vi "Diff_Drive_System_Dash_Write.vi"   [LabVIEW 2019]
uses:
  Diff_Drive_System_Globals.vi
  <vilib>/Rock Robotics/Network Tables/NT Write Numeric Array.vi
  <vilib>/Rock Robotics/Network Tables/NT Write Number.vi
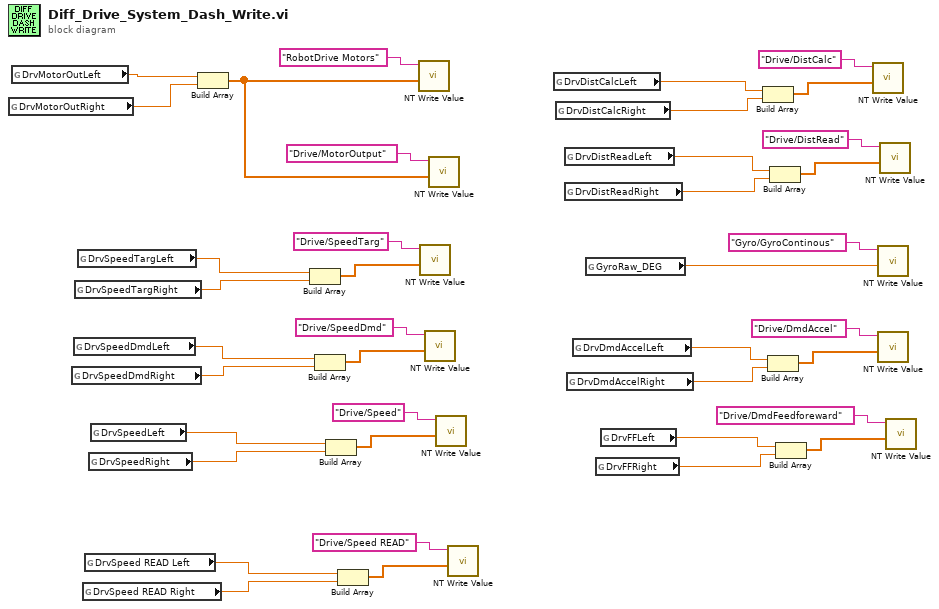
[diagram p0: block diagram]
diagram:
  n1 = global read "Diff_Drive_System_Globals.vi" "DrvMotorOutRight"() -> (w21:dbl)
  n2 = global read "Diff_Drive_System_Globals.vi" "DrvMotorOutLeft"() -> (w22:dbl)
  n3 = global read "Diff_Drive_System_Globals.vi" "DrvSpeedDmdRight"() -> (w16:dbl)
  n4 = global read "Diff_Drive_System_Globals.vi" "DrvSpeedDmdLeft"() -> (w17:dbl)
  n5 = global read "Diff_Drive_System_Globals.vi" "DrvSpeedTargRight"() -> (w18:dbl)
  n6 = global read "Diff_Drive_System_Globals.vi" "DrvSpeedTargLeft"() -> (w19:dbl)
  n7 = global read "Diff_Drive_System_Globals.vi" "DrvSpeed READ Right"() -> (w1:dbl)
  n8 = global read "Diff_Drive_System_Globals.vi" "DrvSpeed READ Left"() -> (w2:dbl)
  n9 = global read "Diff_Drive_System_Globals.vi" "DrvSpeedRight"() -> (w14:dbl)
  n10 = global read "Diff_Drive_System_Globals.vi" "DrvSpeedLeft"() -> (w15:dbl)
  n11 = Build Array(w22, w21) -> (w20:dbl[])
  n12 = Build Array(w19, w18) -> (w25:dbl[])
  n13 = Build Array(w17, w16) -> (w27:dbl[])
  n14 = Build Array(w15, w14) -> (w29:dbl[])
  n15 = Build Array(w2, w1) -> (w3:dbl[])
  n16 = call-poly <vilib>:"NT Write Value.vi"("Numeric Array"=w20, "Name"="RobotDrive Motors") -> ()  [unwired: 9 in, 1 out]
  n17 = call-poly <vilib>:"NT Write Value.vi"("Numeric Array"=w25, "Name"="Drive/SpeedTarg") -> ()  [unwired: 9 in, 1 out]
  n18 = call-poly <vilib>:"NT Write Value.vi"("Numeric Array"=w27, "Name"="Drive/SpeedDmd") -> ()  [unwired: 9 in, 1 out]
  n19 = call-poly <vilib>:"NT Write Value.vi"("Numeric Array"=w20, "Name"="Drive/MotorOutput") -> ()  [unwired: 9 in, 1 out]
  n20 = call-poly <vilib>:"NT Write Value.vi"("Numeric Array"=w29, "Name"="Drive/Speed") -> ()  [unwired: 9 in, 1 out]
  n21 = call-poly <vilib>:"NT Write Value.vi"("Numeric Array"=w3, "Name"="Drive/Speed READ") -> ()  [unwired: 9 in, 1 out]
  n22 = global read "Diff_Drive_System_Globals.vi" "DrvDistCalcLeft"() -> (w13:dbl)
  n23 = global read "Diff_Drive_System_Globals.vi" "DrvDistCalcRight"() -> (w12:dbl)
  n24 = global read "Diff_Drive_System_Globals.vi" "DrvDistReadLeft"() -> (w11:dbl)
  n25 = global read "Diff_Drive_System_Globals.vi" "DrvDistReadRight"() -> (w10:dbl)
  n26 = global read "Diff_Drive_System_Globals.vi" "DrvDmdAccelRight"() -> (w7:dbl)
  n27 = global read "Diff_Drive_System_Globals.vi" "DrvDmdAccelLeft"() -> (w8:dbl)
  n28 = global read "Diff_Drive_System_Globals.vi" "GyroRaw_DEG"() -> (w9:dbl)
  n29 = global read "Diff_Drive_System_Globals.vi" "DrvFFRight"() -> (w5:dbl)
  n30 = global read "Diff_Drive_System_Globals.vi" "DrvFFLeft"() -> (w6:dbl)
  n31 = Build Array(w13, w12) -> (w31:dbl[])
  n32 = Build Array(w8, w7) -> (w36:dbl[])
  n33 = Build Array(w11, w10) -> (w33:dbl[])
  n34 = Build Array(w6, w5) -> (w38:dbl[])
  n35 = call-poly <vilib>:"NT Write Value.vi"("Numeric Array"=w31, "Name"="Drive/DistCalc") -> ()  [unwired: 9 in, 1 out]
  n36 = call-poly <vilib>:"NT Write Value.vi"("Numeric"=w9, "Name"="Gyro/GyroContinous") -> ()  [unwired: 9 in, 1 out]
  n37 = call-poly <vilib>:"NT Write Value.vi"("Numeric Array"=w36, "Name"="Drive/DmdAccel") -> ()  [unwired: 9 in, 1 out]
  n38 = call-poly <vilib>:"NT Write Value.vi"("Numeric Array"=w33, "Name"="Drive/DistRead") -> ()  [unwired: 9 in, 1 out]
  n39 = call-poly <vilib>:"NT Write Value.vi"("Numeric Array"=w38, "Name"="Drive/DmdFeedforeward") -> ()  [unwired: 9 in, 1 out]
